vi "Read Scaling Functions.vi"(8 "error in":errorcluster, 11 "Plugin_UI in":refnum<class "Plugin_UI.lvclass">) -> (0 "error out":errorcluster, 2 "Scaling Functions":T1[](array[typedef]), 3 "Plugin_UI out":refnum<class "Plugin_UI.lvclass">)   [LabVIEW 2020, in "Plugin.lvlib" / "Plugin_UI.lvclass"]
doc: "REad Scaling Function."
uses:
  Plugin_UI.lvclass
  builds/Libraries/LabSys Framework.lvlibp/Configuration Storage/Test Configuration/Function Information.ctl
  builds/Libraries/LabSys Framework.lvlibp/Configuration Storage/Test Configuration/Function Constant Value.ctl
  Plugin_UI.lvclass/Plugin_UI.ctl
  builds/Libraries/LabSys Framework.lvlibp/Configuration Storage/Test Configuration/Test Configuration.lvclass
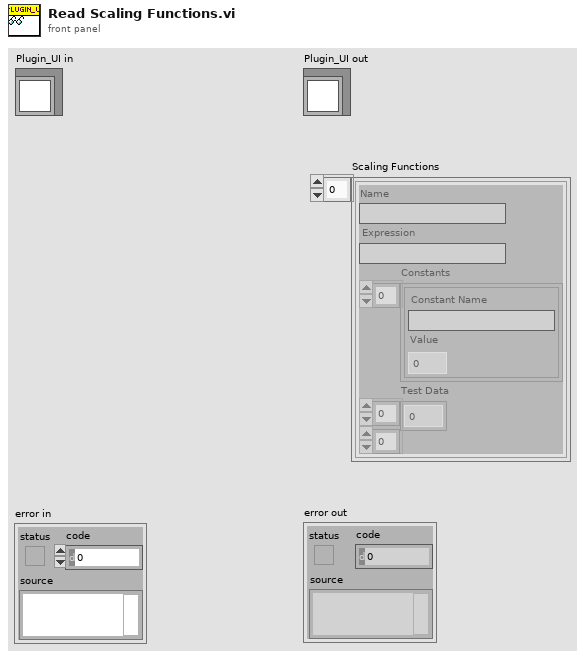
[diagram p1: front panel]
types:
  T1 = typedef "LabSys Framework.lvlibp/Configuration Storage.lvlib/Test Configuration.lvclass/Function Information.ctl" = cluster{"Name":string, "Expression":string, "Constants":T2[], "Test Data":dbl[][]}
  T2 = typedef "LabSys Framework.lvlibp/Configuration Storage.lvlib/Test Configuration.lvclass/Function Constant Value.ctl" = cluster{"Constant Name":string, "Value":dbl}
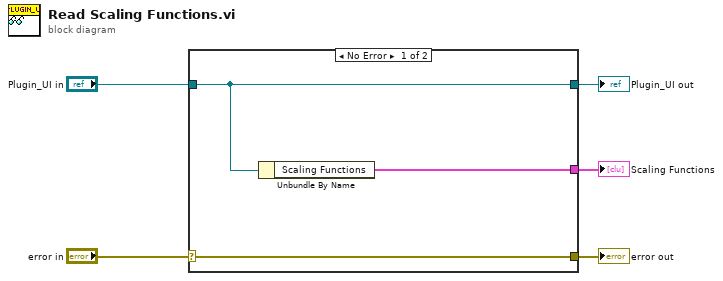
[diagram p0: block diagram]
diagram:
  n1 = case shown="No Error" "error in" {
    selector: "error in" -> [w8 w9]
    tunnel: [w8 w9] -> w4
    tunnel: [w7 w10] -> w2
    tunnel: "Plugin_UI in" -> [w7 w10]
    tunnel: [w6 _] -> w1
    frame No Error {
      n2 = Unbundle By Name(w7) -> ("Scaling Functions"=w6:T1[])
    }
    frame Error {
    }
  }
  "error out" <- w4
  "Plugin_UI out" <- w2
  "Scaling Functions" <- w1
